vi "Read_CubeLiftCommand.vi"(8 "error in (no error)":errorcluster, 11 "CubeLiftData in":refnum<class "CubeLiftData.lvclass">) -> (0 "error out":errorcluster, 2 "Cube Lift Command":T1, 3 "CubeLiftData out":refnum<class "CubeLiftData.lvclass">)   [LabVIEW 2017, in "CubeLiftData.lvclass"]
uses:
  CubeLiftData.lvclass
  Team-code/CubeLiftCommand.ctl
  CubeLiftData.lvclass/CubeLiftData.ctl
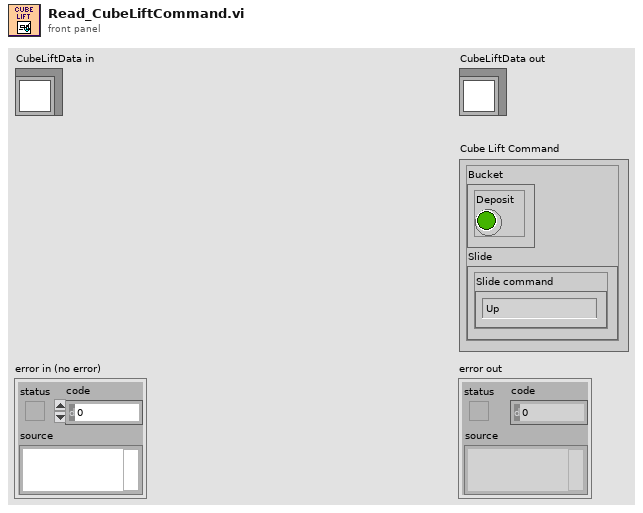
[diagram p1: front panel]
types:
  T1 = typedef "CubeLiftData.lvclass/CubeLiftCommand.ctl" = cluster{"Bucket":cluster{"Deposit":bool}, "Slide":cluster{"Slide command":enum16{"Up", "Down", "Stationary"}}}
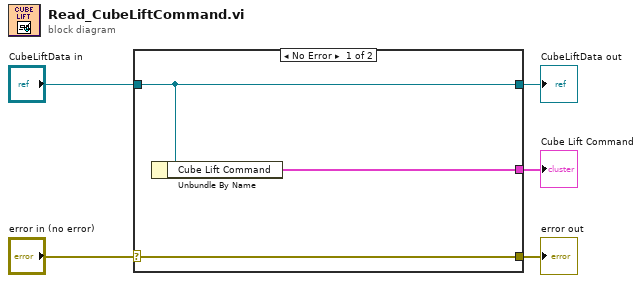
[diagram p0: block diagram]
diagram:
  n1 = case shown="No Error" "error in (no error)" {
    selector: "error in (no error)" -> [w8 w9]
    tunnel: [w8 w9] -> w4
    tunnel: [w7 w10] -> w2
    tunnel: "CubeLiftData in" -> [w7 w10]
    tunnel: [w6 _] -> w1
    frame No Error {
      n2 = Unbundle By Name(w7) -> ("Cube Lift Command"=w6:T1)
    }
    frame Error {
    }
  }
  "error out" <- w4
  "CubeLiftData out" <- w2
  "Cube Lift Command" <- w1
